vi "Cycle End.vi"(8 "error in (no error)":errorcluster, 11 "Plugin Thread in":refnum<class "Plugin Thread.lvclass">) -> (0 "error out":errorcluster, 2 "stop":bool, 3 "Plugin Thread out":refnum<class "Plugin Thread.lvclass">)   [LabVIEW 2019, in "DSF Core.lvlib" / "Plugin Thread.lvclass"]
uses:
  Plugin Thread.lvclass
  C:/Dev/GitHub/niveristand-data-sharing-framework-custom-device/Core/Classes/Thread/Thread.lvclass
  Thread.lvclass
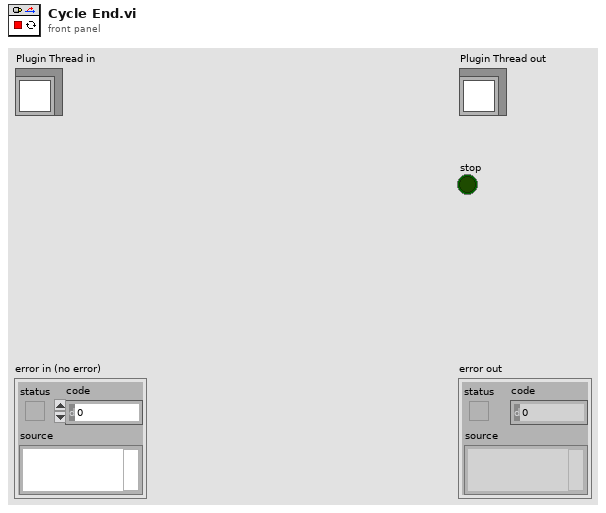
[diagram p1: front panel]
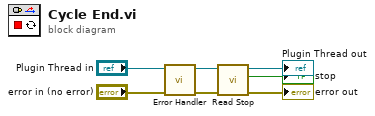
[diagram p0: block diagram]
diagram:
  n1 = call "Error Handler.vi"("error in"="error in (no error)", "plugin thread in"="Plugin Thread in") -> ("error out"=w6:errorcluster, "plugin thread out"=w7:refnum<class "Plugin Thread.lvclass">)  [unwired: 8 in]
  n2 = call "Read Stop.vi"("error in (no error)"=w6, "Thread in"=w7) -> ("error out"=→"error out":errorcluster, "stop"=→"stop":bool, "Thread out"=→"Plugin Thread out":refnum<class "Plugin Thread.lvclass">)  [unwired: 7 in]
